vi "save_device_details.vi"(11 "Device details":T1={"Cell Position"=1, "Cell Label"="", "Pixel to measure"=0, "Area (cm^2)"=0.0919, "Variable"="", "Variable value"="", "Scan settings"=0} {"Pixel to measure" items=["All", "1", "2", "3", "4", "5", "6", "7", "8"]}) -> ()   [LabVIEW 2016]
uses:
  <vilib>/Utility/file.llb/Write Delimited Spreadsheet (string).vi
panel:
  out "error out":errorcluster
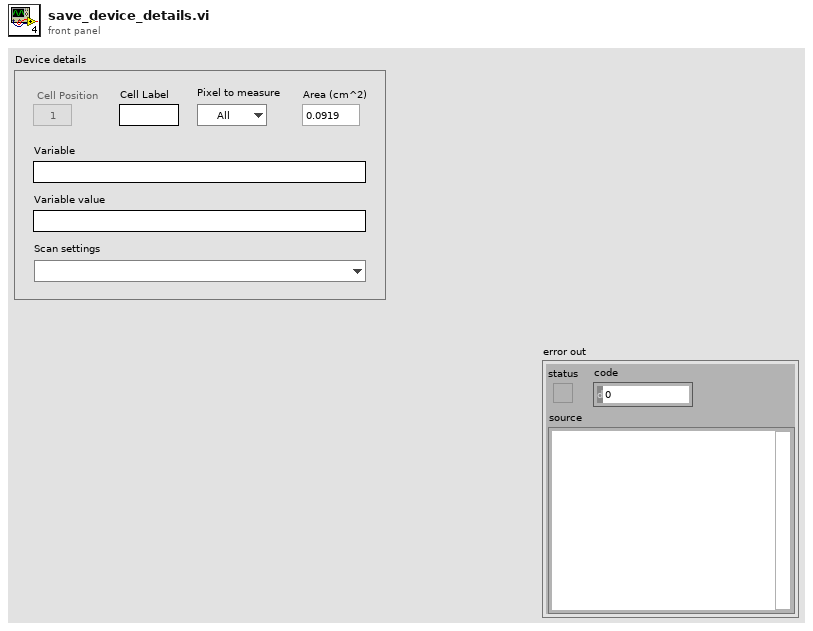
[diagram p1: front panel]
types:
  T1 = cluster{"Cell Position":i32, "Cell Label":string, "Pixel to measure":u16, "Area (cm^2)":dbl, "Variable":string, "Variable value":string, "Scan settings":u16}
  T2 = enum16{"open", "replace", "create", "open or create", "replace or create", "replace or create with confirmation"}
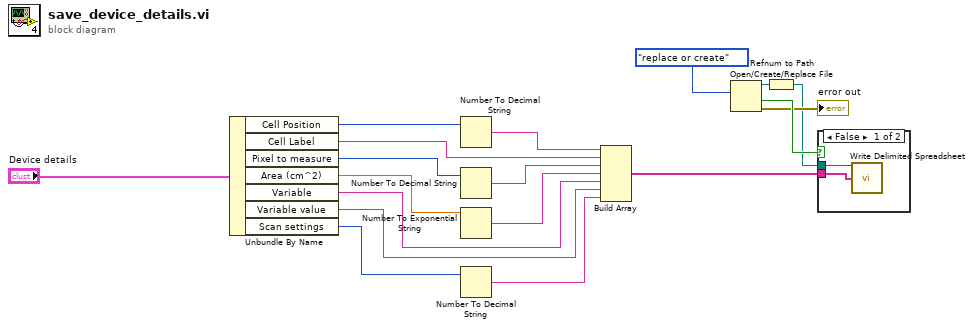
[diagram p0: block diagram]
diagram:
  n1 = Unbundle By Name("Device details") -> ("Cell Position"=w11:i32, "Cell Label"=w6:string, "Pixel to measure"=w10:u16, "Area (cm^2)"=w9:dbl, "Variable"=w3:string, "Variable value"=w2:string, "Scan settings"=w8:u16)
  n2 = Number To Decimal String(number=w11) -> (decimal integer string=w7:string)  [unwired: 1 in]
  n3 = Number To Decimal String(number=w10) -> (decimal integer string=w5:string)  [unwired: 1 in]
  n4 = Number To Exponential String(number=w9) -> (E-format string=w4:string)  [unwired: 3 in]
  n5 = Number To Decimal String(number=w8) -> (decimal integer string=w1:string)  [unwired: 1 in]
  n6 = Build Array(w7, w6, w5, w4, w3, w2, w1) -> (w18:string[])
  n7 = Open/Create/Replace File(operation (0:open)=T2."replace or create") -> (refnum out=w14:refnum<file>, cancelled=w16:bool, error out=→"error out":errorcluster)  [unwired: 5 in]
  n8 = Refnum to Path(1:w14) -> (0:w13:path)
  n9 = case shown="False" w16 {
    tunnel: w18 -> [w19 _]
    tunnel: w13 -> [w20 _]
    frame False {
      n10 = call-poly <vilib>:"Write Delimited Spreadsheet.vi"("file path (dialog if empty)"=w20, "1D data"=w19) -> ()  [unwired: 12 in, 2 out]
    }
    frame True {
    }
  }
